vi "Inst_DS360.vi"(8 "error in":errorcluster, 10 "All Message Queues in":T1, 11 "Prueba07 in":refnum<class "Prueba07.lvclass">) -> (0 "error out":errorcluster)   [LabVIEW 2019, in "Prueba07.lvclass"]
uses:
  Prueba07.lvclass
  QMH/Message Queue/All Message Queues.ctl
  QMH/Message Queue/Message Cluster.ctl
  Prueba07.lvclass/Prueba07.ctl
  ClusterGEN.ctl
  <vilib>/Utility/error.llb/Error Cluster From Error Code.vi
  QMH/Message Queue/Enqueue Message (Single).vi
  <vilib>/ErrorRing/Error Ring.xnode
  QMH/Message Queue/Message Queue.lvlib
  Instrumento/DS360/DS360.lvclass
panel:
  out "All States":string[](array[string])
  out "Actual State":string
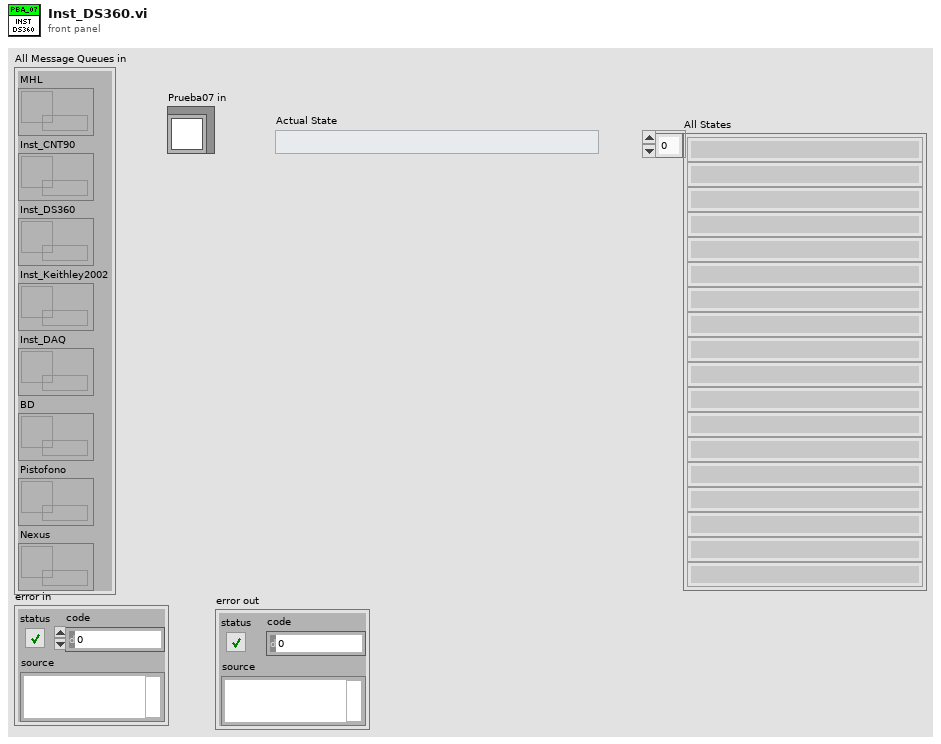
[diagram p1: front panel]
types:
  T1 = typedef "Message Queue.lvlib/All Message Queues.ctl" = cluster{"MHL":refnum<queue>, "Inst_CNT90":refnum<queue>, "Inst_DS360":refnum<queue>, "Inst_Keithley2002":refnum<queue>, "Inst_DAQ":refnum<queue>, "BD":refnum<queue>, "Pistofono":refnum<queue>, "Nexus":refnum<queue>}
  T2 = typedef "Prueba07.lvclass/ClusterGEN.ctl" = cluster{"frec":dbl, "amp":dbl}
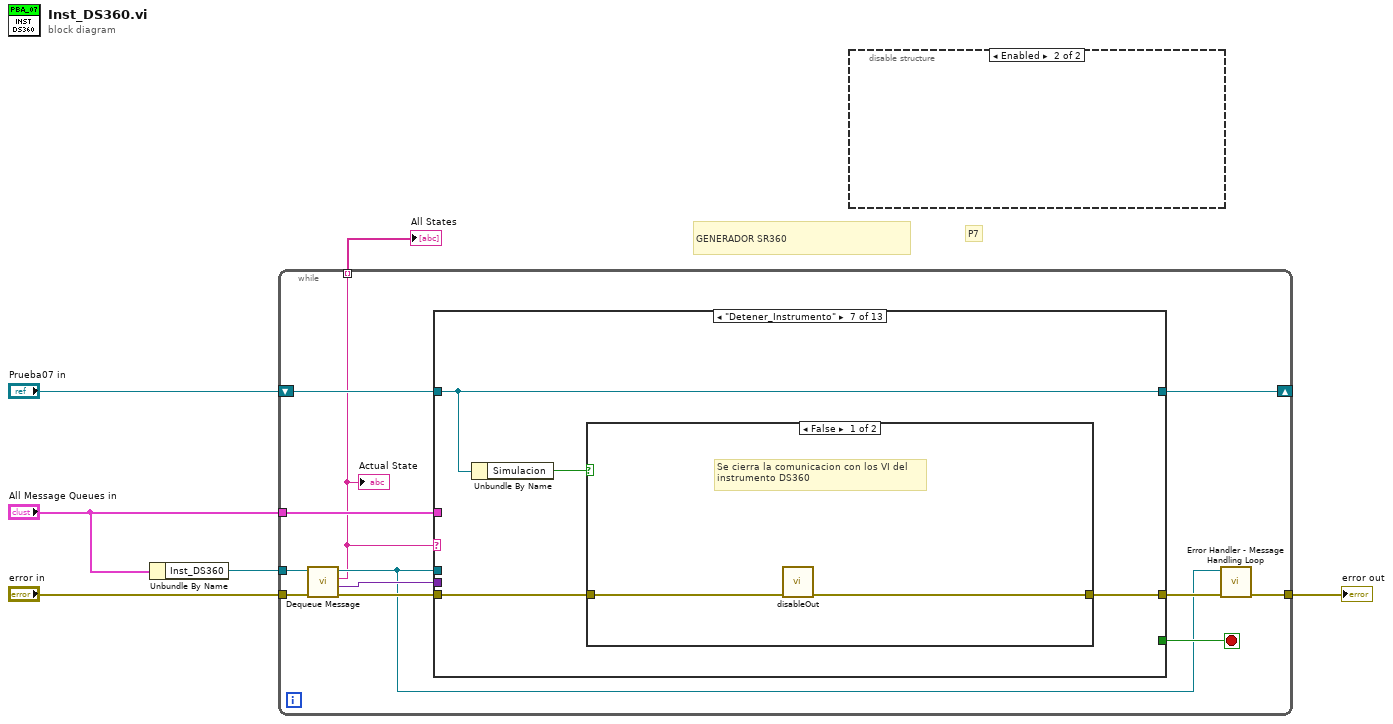
[diagram p0: block diagram]
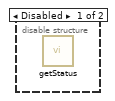
[diagram p2: hidden frame]
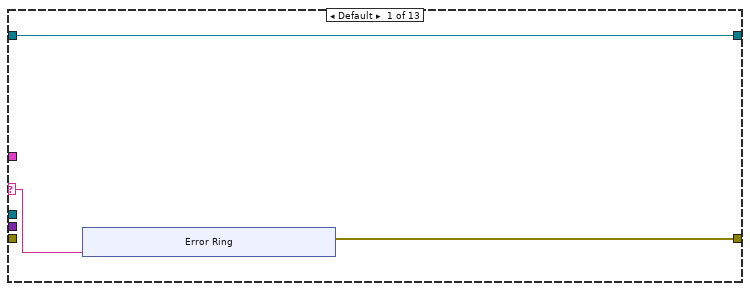
[diagram p3: hidden frame]
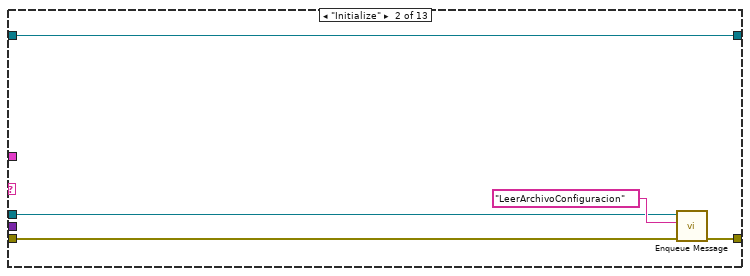
[diagram p4: hidden frame]
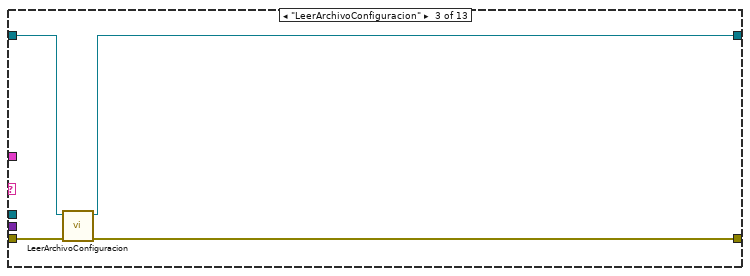
[diagram p5: hidden frame]
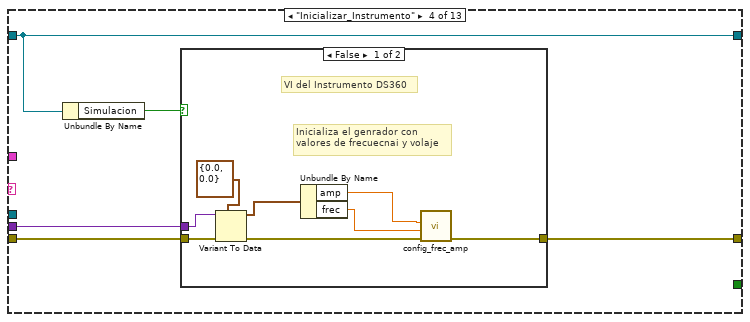
[diagram p6: hidden frame]
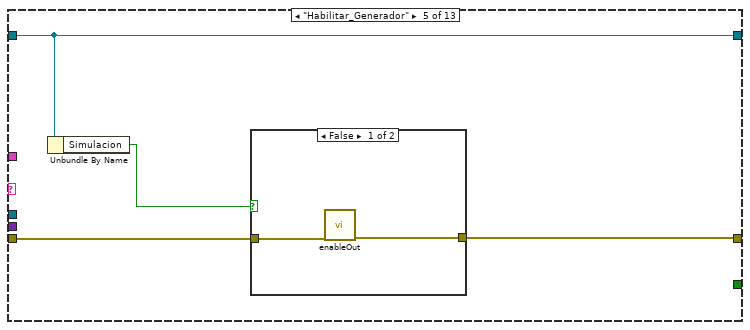
[diagram p8: hidden frame]
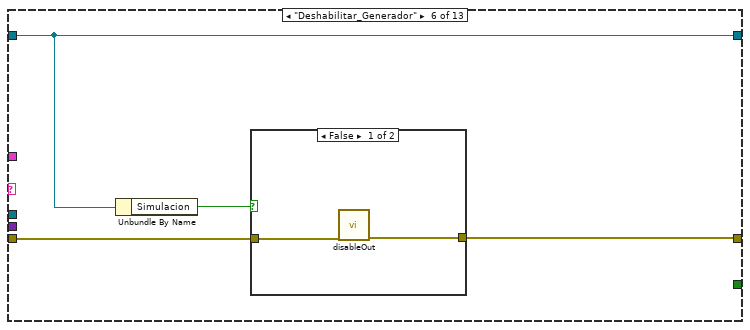
[diagram p10: hidden frame]
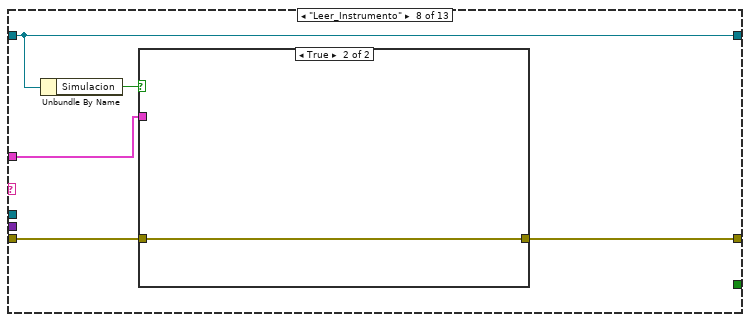
[diagram p13: hidden frame]
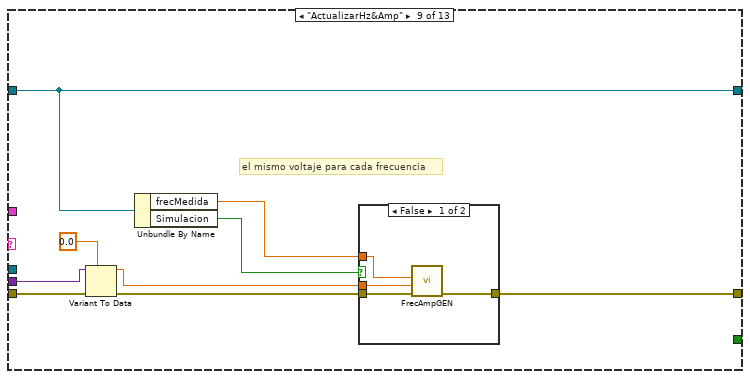
[diagram p15: hidden frame]
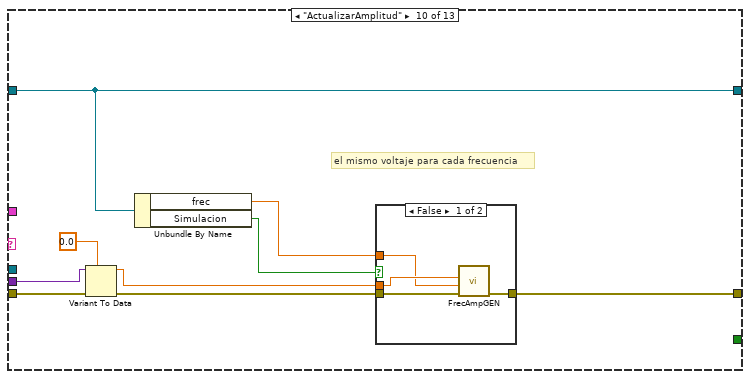
[diagram p17: hidden frame]
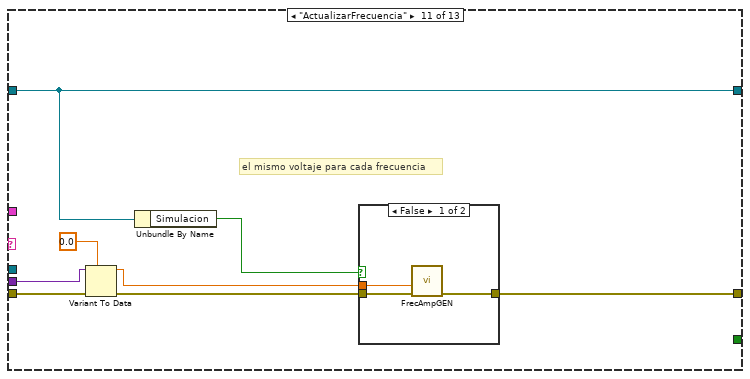
[diagram p19: hidden frame]
diagram:
  # "P7"
  # "GENERADOR SR360"
  n1 = Unbundle By Name("All Message Queues in") -> ("Inst_DS360"=w4:refnum<queue>)
  n2 = while {
    tunnel: "error in" -> [w18]
    tunnel: w4 -> [w17]
    tunnel: "All Message Queues in" -> [w16]
    tunnel: [w9] -> w2
    shift-right: [w12] -> _
    shift-left: "Prueba07 in" -> [w15]
    tunnel: [w7] -> w1 mode=indexing
    stop <- w11 stop-if-true
    n3 = call "Dequeue Message.vi"("error in (no error)"=w18, "Message Queue"=w17) -> ("error out"=w13:errorcluster, "Message Data"=w14:variant, "Message"=w7:string, "dup Message Queue"=w8:refnum<queue>)  [unwired: 6 in]
    "Actual State" <- w7
    n4 = case shown="\"Detener_Instrumento\"" w7 {
      selector: w7 -> [w21 _ _ _ _ _ _ _ _ _ _ w122 _]
      tunnel: w16 -> [_ _ _ _ _ _ _ w76 _ _ _ w121 _]
      tunnel: w15 -> [w19 w33 w34 w40 w53 w60 w68 w75 w84 w95 w111 w129 w131]
      tunnel: w8 -> [_ w29 _ _ _ _ _ _ _ _ _ _ w133]
      tunnel: w14 -> [_ _ _ w39 _ _ _ _ w85 w101 w112 w126 _]
      tunnel: w13 -> [_ w30 w36 w38 w55 w62 w66 w77 w86 w102 w113 w127 w134]
      tunnel: [w20 w31 w37 w42 w54 w61 w69 w73 w88 w94 w115 w124 w130] -> w10
      tunnel: [w19 w33 w35 w40 w53 w60 w68 w75 w84 w95 w111 w129 w131] -> w12
      tunnel: [_ _ _ _ _ _ _ _ _ _ _ _ TRUE] -> w11
      frame Default {
        n5 = xnode "Error Ring"("parameter 0"=w21) -> ("error out"=w20:errorcluster)
      }
      frame "Initialize" {
        n6 = call-poly "Enqueue Message.vi"("error in (no error)"=w30, "Message"="LeerArchivoConfiguracion", "Message Queue"=w29) -> ("error out"=w31:errorcluster)  [unwired: 7 in, 1 out]
      }
      frame "LeerArchivoConfiguracion" {
        n7 = call "LeerArchivoConfiguracion.vi"("error in"=w36, "Prueba07 in"=w34) -> ("error out"=w37:errorcluster, "Prueba07 out"=w35:refnum<class "Prueba07.lvclass">)  [unwired: 8 in]
      }
      frame "Inicializar_Instrumento" {
        n8 = Unbundle By Name(w40) -> ("Simulacion"=w41:bool)
        n9 = case shown="False" w41 {
          tunnel: [w43 w51] -> w42
          tunnel: w38 -> [w50 w51]
          tunnel: w39 -> [w48 _]
          frame False {
            # "Inicializa el genrador con \nvalores de frecuecnai y volaje"
            # "VI del Instrumento DS360"
            n10 = Variant To Data(error in=w50, type=T2 {"frec"=0.0, "amp"=0.0} ("clusterGEN"), Variant=w48) -> (data=w47:T2, error out=w49:errorcluster)
            n11 = Unbundle By Name(w47) -> ("amp"=w46:dbl, "frec"=w45:dbl)
            n12 = call "config_frec_amp.vi"("error in (no error)"=w49, "Frec (Hz)"=w45, "Amplitud (Vrms)"=w46) -> ("error out"=w43:errorcluster)  [unwired: 7 in, 1 out]
          }
          frame True {
            # "Simulacion"
          }
        }
      }
      frame "Habilitar_Generador" {
        n13 = Unbundle By Name(w53) -> ("Simulacion"=w52:bool)
        n14 = case shown="False" w52 {
          tunnel: w55 -> [w57 w58]
          tunnel: [w56 w58] -> w54
          frame False {
            n15 = call "enableOut.vi"("error in (no error)"=w57) -> ("error out"=w56:errorcluster)  [unwired: 9 in, 1 out]
          }
          frame True {
          }
        }
      }
      frame "Deshabilitar_Generador" {
        n16 = Unbundle By Name(w60) -> ("Simulacion"=w59:bool)
        n17 = case shown="False" w59 {
          tunnel: w62 -> [w64 w65]
          tunnel: [w63 w65] -> w61
          frame False {
            n18 = call "disableOut.vi"("error in (no error)"=w64) -> ("error out"=w63:errorcluster)  [unwired: 9 in, 1 out]
          }
          frame True {
          }
        }
      }
      frame "Detener_Instrumento" {
        n19 = Unbundle By Name(w68) -> ("Simulacion"=w67:bool)
        n20 = case shown="False" w67 {
          tunnel: [w71 w72] -> w69
          tunnel: w66 -> [w70 w72]
          frame False {
            # "Se cierra la comunicacion con los VI del\ninstrumento DS360"
            n21 = call "disableOut.vi"("error in (no error)"=w70) -> ("error out"=w71:errorcluster)  [unwired: 9 in, 1 out]
          }
          frame True {
            # "Simulacion"
          }
        }
      }
      frame "Leer_Instrumento" {
        n22 = Unbundle By Name(w75) -> ("Simulacion"=w74:bool)
        n23 = case shown="True" w74 {
          tunnel: [w78 w79] -> w73
          tunnel: w77 -> [w78 w79]
          tunnel: w76 -> [_ _]
          frame False {
          }
          frame True {
          }
        }
      }
      frame "ActualizarHz&Amp" {
        # "el mismo voltaje para cada frecuencia"
        n24 = Variant To Data(error in=w86, type=0.0, Variant=w85) -> (data=w81:dbl, error out=w87:errorcluster)
        n25 = Unbundle By Name(w84) -> ("frecMedida"=w83:dbl, "Simulacion"=w80:bool)
        n26 = case shown="False" w80 {
          tunnel: [w92 w93] -> w88
          tunnel: w87 -> [w91 w93]
          tunnel: w83 -> [w90 _]
          tunnel: w81 -> [w89 _]
          frame False {
            n27 = call "FrecAmpGEN.vi"("error in (no error)"=w91, "Frec (Hz)"=w89, "Amplitud (Vrms)"=w90) -> ("error out"=w92:errorcluster)  [unwired: 7 in, 1 out]
          }
          frame True {
            # "Simlacion"
          }
        }
      }
      frame "ActualizarAmplitud" {
        # "el mismo voltaje para cada frecuencia"
        n28 = Variant To Data(error in=w102, type=0.0, Variant=w101) -> (data=w96:dbl, error out=w97:errorcluster)
        n29 = Unbundle By Name(w95) -> ("frec"=w98:dbl, "Simulacion"=w99:bool)
        n30 = case shown="False" w99 {
          tunnel: [w106 w107] -> w94
          tunnel: w97 -> [w105 w107]
          tunnel: w96 -> [w104 _]
          tunnel: w98 -> [w103 _]
          frame False {
            n31 = call "FrecAmpGEN.vi"("error in (no error)"=w105, "Frec (Hz)"=w103, "Amplitud (Vrms)"=w104) -> ("error out"=w106:errorcluster)  [unwired: 7 in, 1 out]
          }
          frame True {
            # "Simlacion"
          }
        }
      }
      frame "ActualizarFrecuencia" {
        # "el mismo voltaje para cada frecuencia"
        n32 = Variant To Data(error in=w113, type=0.0, Variant=w112) -> (data=w109:dbl, error out=w114:errorcluster)
        n33 = Unbundle By Name(w111) -> ("Simulacion"=w108:bool)
        n34 = case shown="False" w108 {
          tunnel: [w118 w119] -> w115
          tunnel: w114 -> [w117 w119]
          tunnel: w109 -> [w116 _]
          frame False {
            n35 = call "FrecAmpGEN.vi"("error in (no error)"=w117, "Frec (Hz)"=w116) -> ("error out"=w118:errorcluster)  [unwired: 8 in, 1 out]
          }
          frame True {
            # "Simlacion"
          }
        }
      }
      frame "Error" {
        n36 = Unbundle By Name(w121) -> ("MHL"=w120:refnum<queue>)
        n37 = Variant To Data(error in=w127, type=errorcluster {"status"=FALSE, "code"=0, "source"=""} ("error constant"), Variant=w126) -> (data=w123:errorcluster, error out=w125:errorcluster)
        n38 = call-poly "Enqueue Message.vi"("error in (no error)"=w125, "Message Data"=w123, "Message"=w122, "Message Queue"=w120) -> ("error out"=w124:errorcluster)  [unwired: 6 in, 1 out]
      }
      frame "Exit" {
        n39 = Release Queue(queue=w133, error in (no error)=w134) -> (error out=w130:errorcluster)  [unwired: 1 in, 2 out]
      }
    }
    n40 = call "Error Handler - Message Handling Loop.vi"("error in (no error)"=w10, "Message Queue"=w8) -> ("dup error in"=w9:errorcluster)  [unwired: 8 in, 1 out]
  }
  "error out" <- w2
  "All States" <- w1
  n41 = disable-structure shown="Enabled" {
    frame Disabled {
      n42 = call "getStatus.vi"() -> ()  [unwired: 9 in, 3 out]
    }
    frame Enabled {
    }
  }
